vi "SC TCP SoundCheck Control - Exit Soundcheck.vi"(8 "error in (no error)":errorcluster, 11 "TCP Network Connection in":refnum<k5>) -> (0 "error out":errorcluster, 3 "TCP Network Connection out":refnum<k5>)   [LabVIEW 2018]
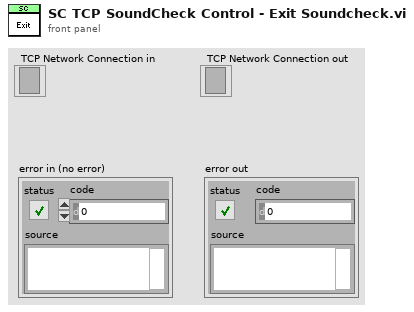
[diagram p1: front panel]
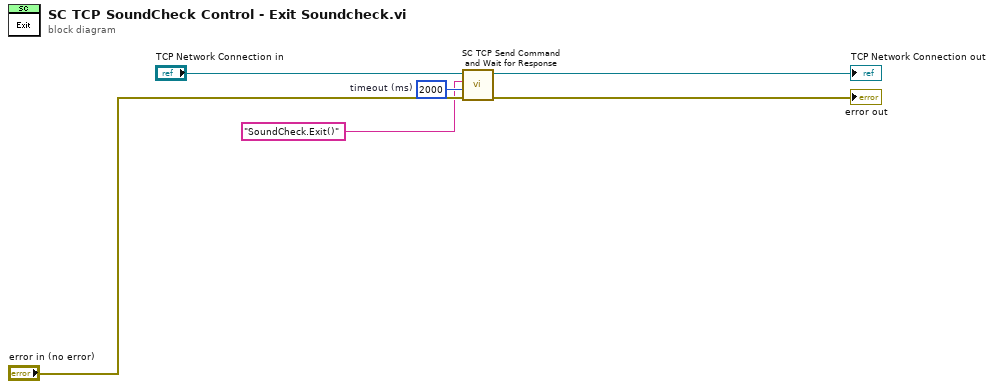
[diagram p0: block diagram]
diagram:
  w3 = 2000  # timeout (ms)
  n1 = call "SC TCP Send Command and Wait for Response.vi"("error in (no error)"="error in (no error)", "timeout (10000 ms)"=w3, "Command"="SoundCheck.Exit()", "TCP Network Connection in"="TCP Network Connection in") -> ("error out"=→"error out":errorcluster, "TCP Network Connection out"=→"TCP Network Connection out":refnum<k5>)  [unwired: 4 in, 2 out]
